vi "Clear XML Dependencies.vi"(8 "error in (no error)":errorcluster, 11 "Project XML Editor in":refnum<class "Project XML Editor.lvclass">) -> (0 "error out":errorcluster, 3 "Project XML Editor out":refnum<class "Project XML Editor.lvclass">)   [LabVIEW 2018, in ".LVLIBP CD XML Updater.lvlib" / "Project XML Editor.lvclass"]
uses:
  Project XML Editor.lvclass
  <vilib>/xml/Close Reference(Node).vi
  <resource>/objmgr/DOMUserDefRef.rc
  <vilib>/xml/NI_XML.lvlib
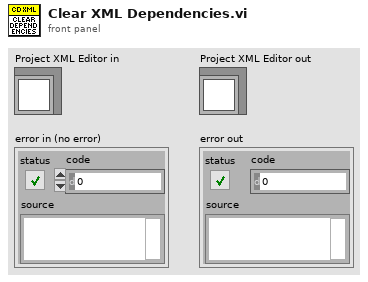
[diagram p1: front panel]
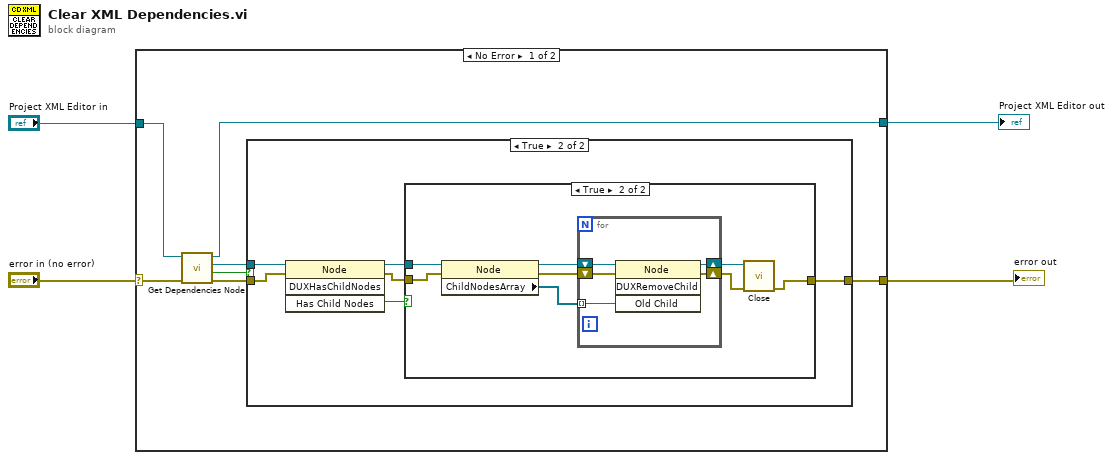
[diagram p0: block diagram]
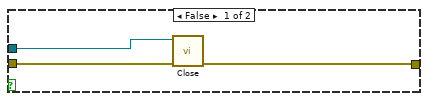
[diagram p3: hidden frame]
diagram:
  n1 = case shown="No Error" "error in (no error)" {
    selector: "error in (no error)" -> [w7 w35]
    tunnel: [w11 w35] -> w4
    tunnel: [w10 w36] -> w3
    tunnel: "Project XML Editor in" -> [w8 w36]
    frame No Error {
      n2 = call "Get Dependencies Node.vi"("error in (no error)"=w7, "Project XML Editor in"=w8) -> ("error out"=w9:errorcluster, "Found?"=w5:bool, "Dependencies out"=w6:refnum<k20>, "Project XML Editor out"=w10:refnum<class "Project XML Editor.lvclass">)  [unwired: 6 in]
      n3 = case shown="True" w5 {
        tunnel: [w12 w18] -> w11
        tunnel: w9 -> [w12 w14]
        tunnel: w6 -> [_ w13]
        frame False {
        }
        frame True {
          n4 = invoke class="Node" method="DUXHasChildNodes"(reference=w13, error in=w14) -> (reference out=w17:refnum<k20>, error out=w16:errorcluster, "Has Child Nodes"=w15:bool)  [unwired: 2 in, 1 out]
          n5 = case shown="True" w15 {
            tunnel: w16 -> [w21 w29]
            tunnel: w17 -> [w20 w26]
            tunnel: [w19 w22] -> w18
            frame False {
              n6 = call-poly <vilib>:"Close.vi"("error in (no error)"=w21, "node"=w20) -> ("error out"=w19:errorcluster)  [unwired: 7 in]
            }
            frame True {
              n7 = property class="Node"(reference=w26, error in=w29) -> (reference out=w27:refnum<k20>, error out=w24:errorcluster, "ChildNodesArray"=w28:refnum<k20>[])
              n8 = for {
                tunnel: w28 -> [w30] mode=indexing
                shift-right: [w33] -> w25
                shift-left: w27 -> [w34]
                shift-right: [w31] -> w23
                shift-left: w24 -> [w32]
                n9 = invoke class="Node" method="DUXRemoveChild"(reference=w34, error in=w32, "Old Child"=w30) -> (reference out=w33:refnum<k20>, error out=w31:errorcluster)  [unwired: 1 in, 2 out]
              }
              n10 = call-poly <vilib>:"Close.vi"("error in (no error)"=w23, "node"=w25) -> ("error out"=w22:errorcluster)  [unwired: 7 in]
            }
          }
        }
      }
    }
    frame Error {
    }
  }
  "error out" <- w4
  "Project XML Editor out" <- w3
